vi "Periodic Tasks.vi"(8 "error in":errorcluster) -> ()   [LabVIEW 2018]
doc: "This VI runs in parallel to other tasks. It can contain as many user-defined periodic loops as you need. These can carry out PID or other sorts of timed response."
uses:
  Left Motors.ctl
  Right Motors.ctl
  Solenoid.ctl
  <vilib>/Rock Robotics/WPI/Solenoid/WPI_SolenoidValue.ctl
  Robot Global Data.vi
  <vilib>/Rock Robotics/WPI/Solenoid/WPI_SolenoidSetEnum.vi
  HuskieLibrary/SwerveLibrary--need to sort/Huskie Swerve.lvlib
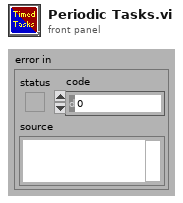
[diagram p1: front panel]
types:
  T1 = typedef "Solenoid.ctl" = enum16{"Solenoid 1", "Solenoid 2", "Solenoid 3", "Solenoid 4"}
  T2 = typedef "Right Motors.ctl" = enum16{"Right Motor 1", "Right Motor 2", "Right Motor 3"}
  T3 = typedef "Left Motors.ctl" = enum16{"Left Motor 1", "Left Motor 2", "Left Motor 3"}
  T4 = typedef "WPI_SolenoidDevRef.ctl" = cluster{"DevStatus":errorcluster, "Pneumatics Control Module":u8, "Forward Solenoid Channel":T5, "Reverse Solenoid Channel":T5}
  T5 = typedef "WPI_SolenoidChannel.ctl" = enum8{"Solenoid 0", "Solenoid 1", "Solenoid 2", "Solenoid 3", "Solenoid 4", "Solenoid 5", "Solenoid 6", "Solenoid 7", "Invalid"}
  T6 = typedef "WPI_MotorControlDeviceRef.ctl" = cluster{"DeviceStatus":errorcluster, "Type":T7, "PWM":cluster{"PWM Channel":T8, "DeadBand":T9}, "CAN":cluster{"Device Number":u8, "SetOutput VI Ref":variant, "GetOutput VI Ref":variant, "Enable VI Ref":variant, "Disable VI Ref":variant, "Data":variant}, "Invert":bool, "DIO PWM":cluster{"PWM \"Enable\" Channel":T8, "DIOChannel":T10, "PWM Rate":dbl}}
  T7 = typedef "WPI_MotorControlType.ctl" = enum16{"PWM", "CAN", "DIO PWM"}
  T8 = typedef "FPGA_DIOPWMChannel.ctl" = enum8{"PWM 0", "PWM 1", "PWM 2", "PWM 3", "PWM 4", "PWM 5", "PWM 6", "PWM 7", "PWM 8", "PWM 9", "PWM MXP 0", "PWM MXP 1", "PWM MXP 2", "PWM MXP 3", "PWM MXP 4", "PWM MXP 5", "PWM MXP 6", "PWM MXP 7", "PWM MXP 8", "PWM MXP 9", "Invalid"}
  T9 = typedef "WPI_PWMDeadband.ctl" = cluster{"Name":string, "maxPositivePwm":i32, "minPositivePwm":i32, "centerPwm":i32, "maxNegativePwm":i32, "minNegativePwm":i32, "angularRange":u16}
  T10 = typedef "FPGA_DIOChannel.ctl" = enum8{"DIO 0", "DIO 1", "DIO 2", "DIO 3", "DIO 4", "DIO 5", "DIO 6", "DIO 7", "DIO 8", "DIO 9", "DIO MXP 0", "DIO MXP 1", "DIO MXP 2", "DIO MXP 3", "DIO MXP 4", "DIO MXP 5", "DIO MXP 6", "DIO MXP 7", "DIO MXP 8", "DIO MXP 9", "DIO MXP 10", "DIO MXP 11", "DIO MXP 12", "DIO MXP 13", "DIO MXP 14", "DIO MXP 15", "SPI Port CS1", "SPI Port CS2", "SPI Port CS3", "SPI Port MISO", "SPI Port MOSI", "Invalid"}
  T11 = typedef "WPI_SolenoidValue.ctl" = enum16{"Off", "On", "Forward", "Reverse"}
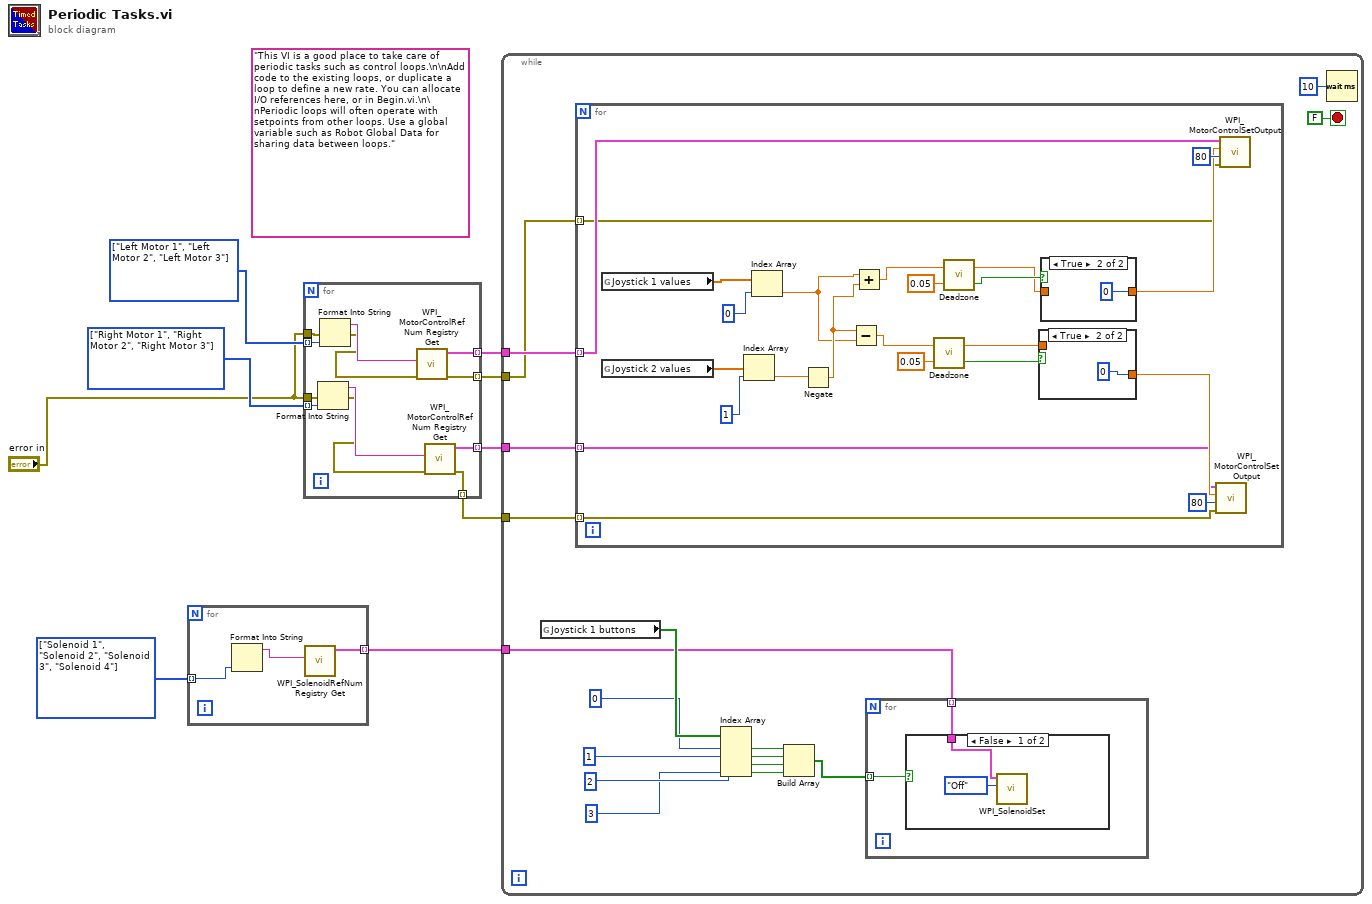
[diagram p0: block diagram]
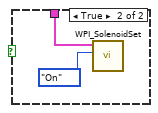
[diagram p2: hidden frame]
diagram:
  w2 = T1[] [enum."Solenoid 1", enum."Solenoid 2", enum."Solenoid 3", enum."Solenoid 4"] items=["Solenoid 1", "Solenoid 2", "Solenoid 3", "Solenoid 4"]
  w8 = T2[] [enum."Right Motor 1", enum."Right Motor 2", enum."Right Motor 3"] items=["Right Motor 1", "Right Motor 2", "Right Motor 3"]
  w9 = T3[] [enum."Left Motor 1", enum."Left Motor 2", enum."Left Motor 3"] items=["Left Motor 1", "Left Motor 2", "Left Motor 3"]
  (unwired) "This VI is a good place to take care of periodic tasks such as control loops.\n\nAdd code to the existing loops, or duplicate a loop to define a new rate. You can allocate I/O references here, or in Begin.vi.\n\nPeriodic loops will often operate with setpoints from other loops. Use a global variable such as Robot Global Data for sharing data between loops."
  n1 = for {
    tunnel: w2 -> [w11] mode=indexing
    tunnel: [w10] -> w1 mode=indexing
    n2 = Format Into String(w11) -> (resulting string=w12:string)  [unwired: 3 in, 1 out]
    n3 = call <vilib>:"WPI_SolenoidRefNum Registry Get.vi"("refnum name"=w12) -> ("SolenoidDevRef"=w10:T4)  [unwired: 9 in, 1 out]
  }
  n4 = for {
    tunnel: w9 -> [w24] mode=indexing
    tunnel: w8 -> [w21] mode=indexing
    tunnel: "error in" -> [w20]
    tunnel: "error in" -> [w19]
    tunnel: [w16] -> w6 mode=indexing
    tunnel: [w15] -> w5 mode=indexing
    tunnel: [w14] -> w4 mode=indexing
    tunnel: [w13] -> w3 mode=indexing
    n5 = Format Into String(error in=w20, w21) -> (resulting string=w22:string, error out=w17:errorcluster)  [unwired: 2 in]
    n6 = Format Into String(error in=w19, w24) -> (resulting string=w23:string, error out=w18:errorcluster)  [unwired: 2 in]
    n7 = call <vilib>:"WPI_MotorControlRefNum Registry Get.vi"("error in (no error)"=w18, "refnum name"=w23) -> ("error out"=w13:errorcluster, "MotorControlDevRef"=w16:T6)  [unwired: 8 in]
    n8 = call <vilib>:"WPI_MotorControlRefNum Registry Get.vi"("error in (no error)"=w17, "refnum name"=w22) -> ("error out"=w14:errorcluster, "MotorControlDevRef"=w15:T6)  [unwired: 8 in]
  }
  n9 = while {
    tunnel: w6 -> [w39]
    tunnel: w5 -> [w38]
    tunnel: w4 -> [w37]
    tunnel: w3 -> [w36]
    tunnel: w1 -> [w26]
    stop <- FALSE stop-if-true
    n10 = global read "Robot Global Data.vi" "Joystick 1 buttons"() -> (w35:bool[])
    n11 = for {
      tunnel: w39 -> [w60] mode=indexing
      tunnel: w38 -> [w58] mode=indexing
      tunnel: w37 -> [w57] mode=indexing
      tunnel: w36 -> [w56] mode=indexing
      n12 = global read "Robot Global Data.vi" "Joystick 1 values"() -> (w70:dbl[])
      n13 = global read "Robot Global Data.vi" "Joystick 2 values"() -> (w68:dbl[])
      n14 = Index Array(array=w68, index=1) -> (element=w66:dbl)
      n15 = Index Array(array=w70, index=0) -> (element=w64:dbl)
      n16 = Negate(x=w66) -> (-x=w65:dbl)
      n17 = Subtract(x=w65, y=w64) -> (x-y=w55:dbl)
      n18 = Add(x=w64, y=w65) -> (x+y=w54:dbl)
      n19 = call "Deadzone.vi"("Deadzone"=0.05, "Value"=w55) -> ("Inside Deadzone?"=w52:bool, "Numeric"=w50:dbl)
      n20 = call "Deadzone.vi"("Deadzone"=0.05, "Value"=w54) -> ("Inside Deadzone?"=w53:bool, "Numeric"=w51:dbl)
      n21 = case shown="True" w52 {
        tunnel: [w71 0] -> w59
        tunnel: w50 -> [w71 _]
        frame False {
        }
        frame True {
        }
      }
      n22 = case shown="True" w53 {
        tunnel: [w73 0] -> w61
        tunnel: w51 -> [w73 _]
        frame False {
        }
        frame True {
        }
      }
      n23 = call <vilib>:"WPI_MotorControlSetOutput.vi"("error in (no error)"=w57, "options"=u8 80, "Output"=w59, "MotorControlDevRef"=w58) -> ()  [unwired: 5 in, 3 out]
      n24 = call <vilib>:"WPI_MotorControlSetOutput.vi"("error in (no error)"=w56, "options"=u8 80, "Output"=w61, "MotorControlDevRef"=w60) -> ()  [unwired: 5 in, 3 out]
    }
    n25 = Index Array(array=w35, index #1=0 ("index"), index #2=1 ("index"), index #3=2 ("index"), index #4=3 ("index")) -> (element #1=w30:bool, element #2=w29:bool, element #3=w28:bool, element #4=w27:bool)
    n26 = Build Array(w30, w29, w28, w27) -> (w25:bool[])
    n27 = for {
      tunnel: w26 -> [w43] mode=indexing
      tunnel: w25 -> [w42] mode=indexing
      n28 = case shown="False" w42 {
        tunnel: w43 -> [w44 w46]
        frame False {
          n29 = call-poly <vilib>:"WPI_SolenoidSet.vi"("Value"=WPI_SolenoidValue."Off", "SolenoidDevRef"=w44) -> ()  [unwired: 8 in, 2 out]
        }
        frame True {
          n30 = call-poly <vilib>:"WPI_SolenoidSet.vi"("Value"=WPI_SolenoidValue."On", "SolenoidDevRef"=w46) -> ()  [unwired: 8 in, 2 out]
        }
      }
    }
    n31 = Wait (ms)(milliseconds to wait=u32 10) -> ()  [unwired: 1 out]
  }
